vi "CarayaTest.vi"   [LabVIEW 2020]
uses:
  LabVIEW Data/Calculator/Calculator.lvclass
  <vilib>/addons/_JKI Toolkits/Caraya/classes/Assert/Assert True.vi
  <vilib>/addons/_JKI Toolkits/Caraya/classes/Test/Test.lvclass
  <vilib>/addons/_JKI Toolkits/Caraya/classes/Assert/Assert.lvclass
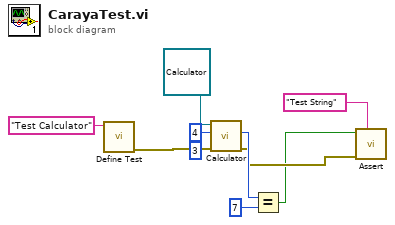
[diagram p0: block diagram]
diagram:
  n1 = call <vilib>:"Define Test.vi"("Label (VI Title)"="Test Calculator") -> ("error out"=w9:errorcluster)  [unwired: 10 in]
  n2 = call "Calculator.vi"("error in (no error)"=w9, "Input 2"=3, "Input 1"=4, "Calculator in"=refnum<class "Calculator.lvclass"> refnum) -> ("error out"=w4:errorcluster, "Output"=w5:i32)  [unwired: 5 in, 1 out]
  n3 = Equal?(x=w5, y=7) -> (x = y?=w2:bool)
  n4 = call-poly <vilib>:"Assert.vi"("Label"="Test String", "error in (no error)"=w4, "True?"=w2) -> ()  [unwired: 8 in, 1 out]
